vi "get img.vi"(8 "error in (no error)":errorcluster caption="Fehler (Eingang, kein Fehler)", 10 "index":i32 caption="Index", 11 "Segment (Eingang)":refnum<class "Segment.lvclass">) -> (0 "error out":errorcluster caption="Fehler (Ausgang)", 2 "img.lvclass":refnum<class "img.lvclass">, 3 "Segment (Ausgang)":refnum<class "Segment.lvclass">)   [LabVIEW 2013, in "DatenKlassen.lvlib" / "Segment.lvclass"]
uses:
  Segment.lvclass
  Image/img.lvclass
  Segment.lvclass/Segment.ctl
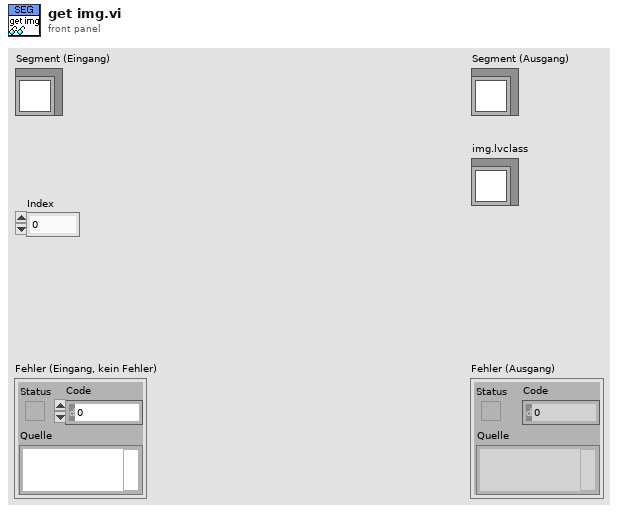
[diagram p1: front panel]
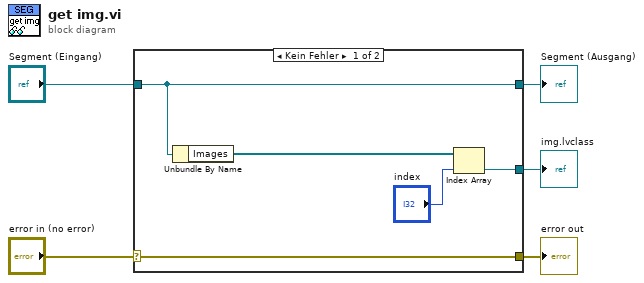
[diagram p0: block diagram]
diagram:
  n1 = case shown="Kein Fehler" "error in (no error)" {
    selector: "error in (no error)" -> [w10 w11]
    tunnel: [w10 w11] -> w4
    tunnel: [w9 w12] -> w2
    tunnel: "Segment (Eingang)" -> [w9 w12]
    tunnel: [w6 _] -> w1
    frame No Error {
      n2 = Unbundle By Name(w9) -> ("Images"=w8:refnum<class "img.lvclass">[])
      n3 = Index Array(array=w8, index="index") -> (element=w6:refnum<class "img.lvclass">)
    }
    frame Error {
    }
  }
  "error out" <- w4
  "Segment (Ausgang)" <- w2
  "img.lvclass" <- w1
